vi "OP400ZP_prep bdd init.vi"(10 "tabin":string[](array[string])) -> (3 "Tableau":string[](array[string]))   [LabVIEW 2020]
uses:
  OP400ZP_selectdata.ctl
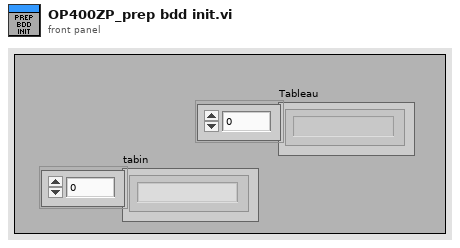
[diagram p1: front panel]
types:
  T1 = typedef "OP400ZP_selectdata.ctl" = u16
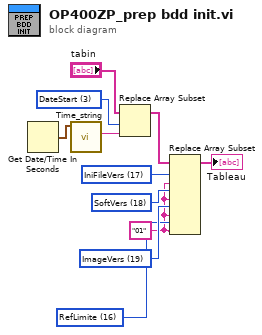
[diagram p0: block diagram]
diagram:
  w2 = T1 16 items=["IdOp400", "SN", "Type", "DateStart", "OCV", "ACIR", "InsuP", "InsuN", "TC0", "TC1", "DeltaTC", "VC0", "VC1", "DeltaVC", "MCU", "Tfactory", "RefLimite", "IniFileVers", "SoftVers", "ImageVers", "Pass", "Operateur", "TempsTest"] ("Menu déroulant")
  w3 = T1 19 items=["IdOp400", "SN", "Type", "DateStart", "OCV", "ACIR", "InsuP", "InsuN", "TC0", "TC1", "DeltaTC", "VC0", "VC1", "DeltaVC", "MCU", "Tfactory", "RefLimite", "IniFileVers", "SoftVers", "ImageVers", "Pass", "Operateur", "TempsTest"] ("Menu déroulant")
  w4 = T1 18 items=["IdOp400", "SN", "Type", "DateStart", "OCV", "ACIR", "InsuP", "InsuN", "TC0", "TC1", "DeltaTC", "VC0", "VC1", "DeltaVC", "MCU", "Tfactory", "RefLimite", "IniFileVers", "SoftVers", "ImageVers", "Pass", "Operateur", "TempsTest"] ("Menu déroulant")
  w5 = T1 17 items=["IdOp400", "SN", "Type", "DateStart", "OCV", "ACIR", "InsuP", "InsuN", "TC0", "TC1", "DeltaTC", "VC0", "VC1", "DeltaVC", "MCU", "Tfactory", "RefLimite", "IniFileVers", "SoftVers", "ImageVers", "Pass", "Operateur", "TempsTest"] ("Menu déroulant")
  w6 = T1 3 items=["IdOp400", "SN", "Type", "DateStart", "OCV", "ACIR", "InsuP", "InsuN", "TC0", "TC1", "DeltaTC", "VC0", "VC1", "DeltaVC", "MCU", "Tfactory", "RefLimite", "IniFileVers", "SoftVers", "ImageVers", "Pass", "Operateur", "TempsTest"] ("Menu déroulant")
  w1 = "01" ("nouvel élément/sous-tableau")
  n1 = Get Date/Time In Seconds() -> (seconds since 1Jan1904=w11:timestamp)
  n2 = call <userlib>:"Time_string.vi"("h in"=w11) -> ("heure sql"=w10:string)  [unwired: 9 in, 1 out]
  n3 = Replace Array Subset(array="tabin", new element=w10, index=w6) -> (w7:string[])
  n4 = Replace Array Subset(array=w7, new element #1=w1, index #1=w5, new element #2=w1, index #2=w4, new element #3=w1, index #3=w3, new element #4=w1, index #4=w2) -> (→"Tableau":string[])
